vi "Test Suite Filter Select Class.vi"(8 "error in (no error)":errorcluster, 11 "Test Case In":refnum<class "LUnit Test Suite Tests.lvclass">) -> (0 "error out":errorcluster, 3 "Test Case Out":refnum<class "LUnit Test Suite Tests.lvclass">)   [LabVIEW 2020, in "LUnit Test Suite Tests.lvclass"]
uses:
  LUnit Test Suite Tests.lvclass
  Test Doubles/Test Case Test Double Child/Light Test Case Double.lvclass
  C:/git/astemes-lunit/source/API/LUnit Test Case/LUnit Test Case.lvclass
  source/API/LUnit Test Suite/LUnit Test Suite.lvclass
  C:/git/astemes-lunit/source/Core/Runnable/Runnable.lvclass
  source/Core/Runnable/Runnable.lvclass
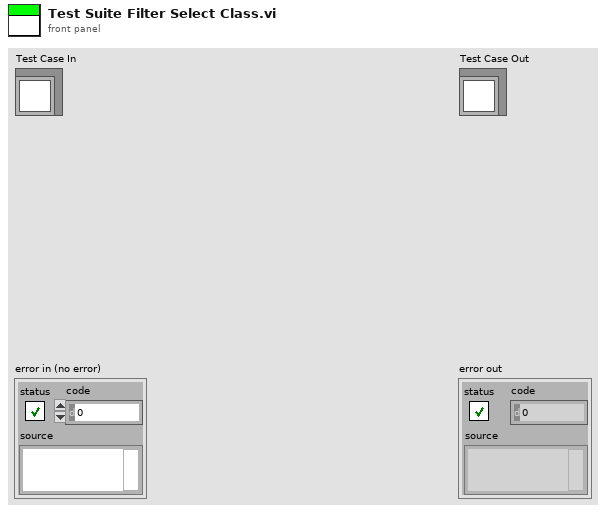
[diagram p1: front panel]
types:
  T1 = typedef "Result.lvlib/Result.ctl" = cluster{"Name":string, "Message":string, "Description":string, "Status":T2, "Result Type":T3, "Execution Time":dbl}
  T2 = typedef "Result.lvlib/Status.ctl" = enum16{"", "Passed", "Failed", "Error", "Skipped", "Setup Error", "Broken", "Teardown Error"}
  T3 = typedef "Result.lvlib/Type.ctl" = enum16{"Method", "Case", "Suite", "Pass", "Fail", "Skip", "Pass if", "Fail if", "Pass if Error", "Fail if Error", "Pass if Equal", "Fail if Equal"}
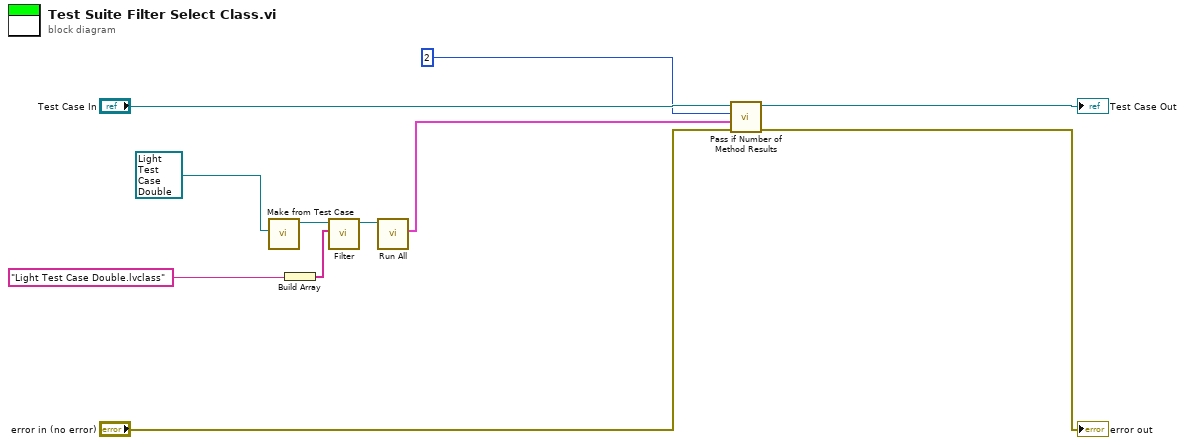
[diagram p0: block diagram]
diagram:
  n1 = call "Make from Test Case.vi"("LUnit Test Case"=refnum<class "Light Test Case Double.lvclass"> refnum ("Light Test Case Double.lvclass")) -> ("LUnit Test Suite Out"=w7:refnum<class "LUnit Test Suite.lvclass">)  [unwired: 9 in, 1 out]
  n2 = Build Array("Light Test Case Double.lvclass" ("Methods")) -> (w3:string[])
  n3 = call-dynamic "Filter.vi"("Selected Runnables"=w3, "LUnit Test Suite In"=w7) -> ("LUnit Test Suite Out"=w5:refnum<class "LUnit Test Suite.lvclass">)  [unwired: 8 in, 1 out]
  n4 = call "Run All.vi"("Runnable In"=w5) -> ("Results"=w2:T1[])  [unwired: 9 in, 1 out]
  n5 = call "Pass if Number of Method Results.vi"("error in (no error)"="error in (no error)", "Results"=w2, "Remaining Results"=2, "LUnit Test Suite Tests in"="Test Case In") -> ("error out"=→"error out":errorcluster, "LUnit Test Suite Tests out"=→"Test Case Out":refnum<class "LUnit Test Suite Tests.lvclass">)  [unwired: 6 in]
